vi "CLD 10 Unbundle data SubVI.vi"(8 "error in (no error)":errorcluster, 10 "Current State Number":i32, 11 "[Data In]":T1[](array[typedef])) -> (0 "error out":errorcluster, 1 "State 3":bool, 2 "State 2":bool, 3 "[Data Out]":T1[](array[typedef]), 4 "Next Dwell Time":dbl, 5 "State 1":bool, 6 "Dwell Time":dbl)   [LabVIEW 2025]
doc: "CLD 10 exercise.\n\nThis SubVI is used to simplify the reading of data from the cluster array in the main application."
uses:
  CLD 10 CSV file data structure.ctl
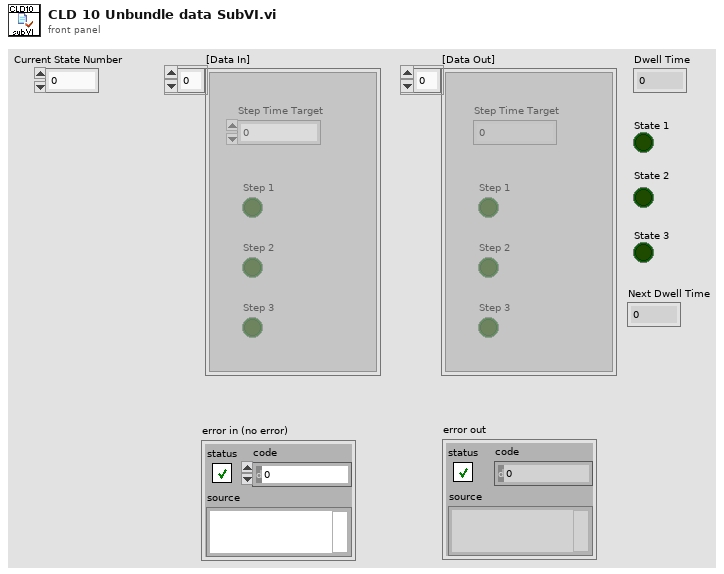
[diagram p1: front panel]
types:
  T1 = typedef "CLD 10 CSV file data structure.ctl" = cluster{"Step Time Target":i32, "Step 1":bool, "Step 2":bool, "Step 3":bool}
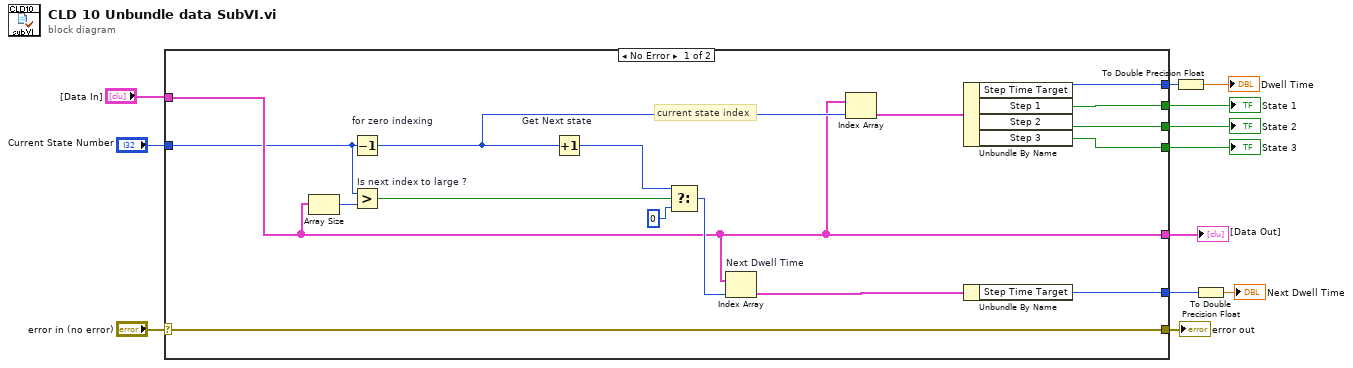
[diagram p0: block diagram]
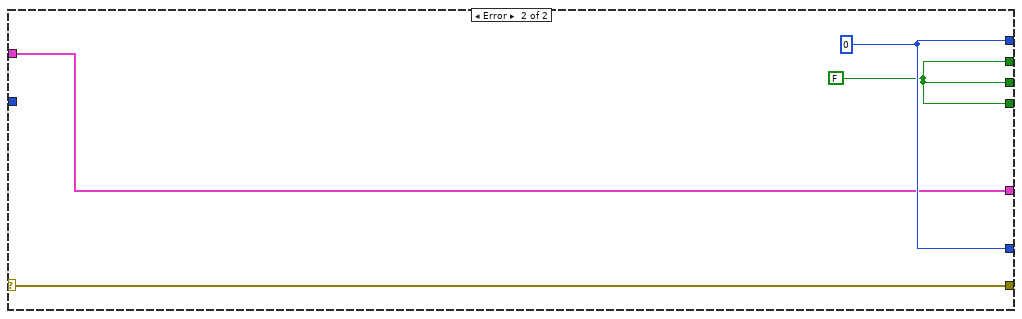
[diagram p2: hidden frame]
diagram:
  n1 = case shown="No Error" "error in (no error)" {
    selector: "error in (no error)" -> [w15 w32]
    tunnel: [w27 w30] -> w12
    tunnel: [w26 w30] -> w11
    tunnel: [w25 w30] -> w10
    tunnel: [w24 w31] -> w9
    tunnel: "[Data In]" -> [w14 w29]
    tunnel: [w17 w31] -> w6
    tunnel: [w15 w32] -> w3
    tunnel: [w14 w29] -> w2
    tunnel: "Current State Number" -> [w13 _]
    frame No Error {
      # "current state index"
      n2 = Array Size(array=w14) -> (size(s)=w20:i32)
      n3 = Decrement "for zero indexing"(x=w13) -> (x-1=w16:i32)
      n4 = Greater? "Is next index to large ?"(x=w13, y=w20) -> (0:w23:bool)
      n5 = Increment "Get Next state"(x=w16) -> (x+1=w19:i32)
      n6 = Select(t=w19, s=w23, f=0) -> (s? t:f=w21:i32)
      n7 = Index Array "Next Dwell Time"(array=w14, index=w21) -> (element=w18:T1)
      n8 = Index Array(array=w14, index=w16) -> (element=w28:T1)
      n9 = Unbundle By Name(w28) -> ("Step Time Target"=w24:i32, "Step 1"=w27:bool, "Step 2"=w26:bool, "Step 3"=w25:bool)
      n10 = Unbundle By Name(w18) -> ("Step Time Target"=w17:i32)
    }
    frame Error {
      w30 = FALSE ("State 1")
      w31 = 0 ("Dwell Time")
    }
  }
  "State 1" <- w12
  "State 2" <- w11
  "State 3" <- w10
  "error out" <- w3
  "[Data Out]" <- w2
  n11 = To Double Precision Float(number=w9) -> (double precision float=→"Dwell Time":dbl)
  n12 = To Double Precision Float(number=w6) -> (double precision float=→"Next Dwell Time":dbl)
